vi "Configure User Parameters.vi"(7 "Currency (0: Dollar)":u16(ring) items=["Dollar", "Euro"], 8 "error in (no error)":errorcluster, 9 "Threshold (0 W)":dbl, 10 "Rate (0.000 $)":dbl, 11 "VISA resource name":refnum<visa-resource-name>) -> (0 "error out":errorcluster, 3 "VISA resource name out":refnum<visa-resource-name>)   [LabVIEW 2013, in "Watts Up Series.lvlib"]
doc: "Configures the rate, threshold and currency type for the Watts Up device."
uses:
  <instrlib>/Watts Up Series/Watts Up Series.lvlib
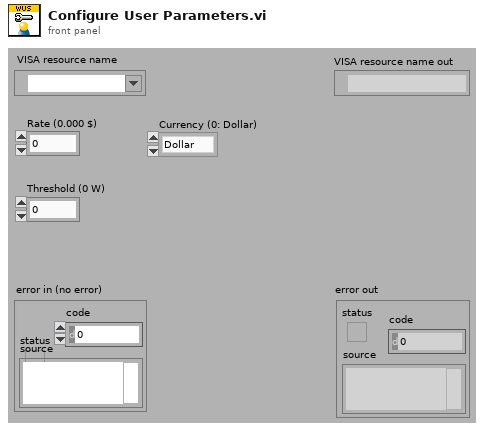
[diagram p1: front panel]
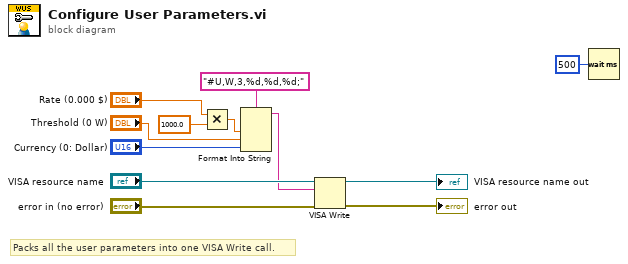
[diagram p0: block diagram]
diagram:
  # "Packs all the user parameters into one VISA Write call."
  n1 = Multiply(x="Rate (0.000 $)", y=1000.0) -> (x*y=w2:dbl)
  n2 = Format Into String(format string="#U,W,3,%d,%d,%d;", w2, "Threshold (0 W)", "Currency (0: Dollar)") -> (resulting string=w5:string)  [unwired: 2 in, 1 out]
  n3 = VISA Write(VISA resource name="VISA resource name", write buffer=w5, error in (no error)="error in (no error)") -> (VISA resource name out=→"VISA resource name out":refnum<visa-resource-name>, error out=→"error out":errorcluster)  [unwired: 1 out]
  n4 = Wait (ms)(milliseconds to wait=u32 500) -> ()  [unwired: 1 out]
